vi "Save images to avi.vi"(4 "Camera 2?":bool, 6 "AVI Refnum 2":T1, 7 "Images Out":T2[](array[typedef]), 9 "Buffer size":i32, 10 "Images Out 2":T2[](array[typedef]), 11 "AVI refnum 1":T1) -> (2 "AVI Refnum 2":T1, 3 "AVI Refnum 1":T1)   [LabVIEW 2018]
uses:
  <vilib>/vision/Avi.llb/IMAQ AVI2 Refnum.ctl
  <vilib>/vision/Image Controls.llb/IMAQ Image.ctl
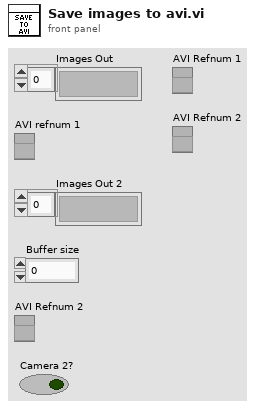
[diagram p1: front panel]
types:
  T1 = typedef "IMAQ AVI2 Refnum.ctl" = refnum<k20>
  T2 = typedef "IMAQ Image.ctl" = refnum<image>
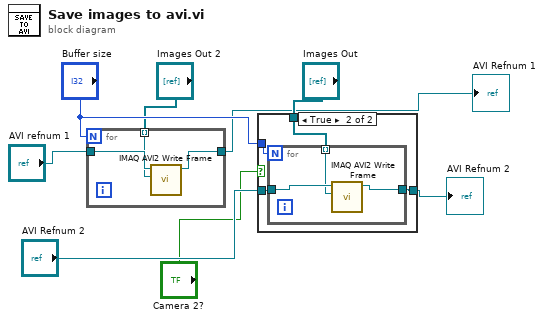
[diagram p0: block diagram]
diagram:
  n1 = for {
    N: "Buffer size" -> [_]
    tunnel: "Images Out 2" -> [w9] mode=indexing
    tunnel: "AVI refnum 1" -> [w11]
    tunnel: [w10] -> w2
    n2 = call "IMAQ AVI2 Write Frame"("Image"=w9, "AVI Refnum"=w11) -> ("AVI Refnum (duplicate)"=w10:T1)  [unwired: 7 in, 2 out]
  }
  "AVI Refnum 1" <- w2
  n3 = case shown="True" "Camera 2?" {
    tunnel: "Images Out" -> [_ w16]
    tunnel: "AVI Refnum 2" -> [w12 w15]
    tunnel: [w12 w14] -> w7
    tunnel: "Buffer size" -> [_ w13]
    frame False {
    }
    frame True {
      n4 = for {
        N: w13 -> [_]
        tunnel: w16 -> [w17] mode=indexing
        tunnel: w15 -> [w19]
        tunnel: [w18] -> w14
        n5 = call "IMAQ AVI2 Write Frame"("Image"=w17, "AVI Refnum"=w19) -> ("AVI Refnum (duplicate)"=w18:T1)  [unwired: 7 in, 2 out]
      }
    }
  }
  "AVI Refnum 2" <- w7
